vi "Setup UI.vi"(8 "error in (no error)":errorcluster, 11 "Operator UI in":refnum<class "Measurement UI.lvclass">) -> (0 "error out":errorcluster, 3 "Operator UI out":refnum<class "Measurement UI.lvclass">)   [LabVIEW 2015, in "Measurement UI.lvlib" / "Measurement UI.lvclass"]
uses:
  Measurement UI.lvclass
  Measurement UI.lvclass/Measurement UI.ctl
  <vilib>/Utility/miscctls.llb/LVRowAndColumnTypeDef.ctl
  <vilib>/Utility/miscctls.llb/LVRowAndColumnUnsignedTypeDef.ctl
  Accessors/Read Show FP_.vi
  Accessors/Read Status Display.vi
  Accessors/Read Digitizer.vi
  Accessors/Read Results Listbox.vi
  Accessors/Read View Results.vi
  Accessors/Read Function Generator.vi
  Accessors/Read Tab Control.vi
  Read Multimeter.vi
  Accessors/Read Run.vi
  Accessors/Read Measurement.vi
  Accessors/Read Power Supply.vi
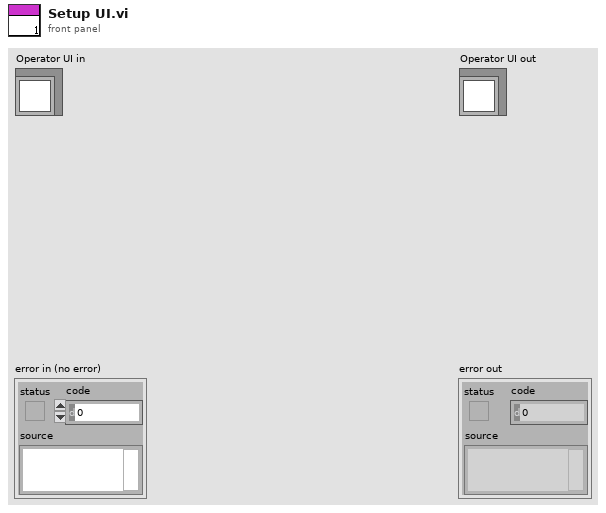
[diagram p1: front panel]
types:
  T1 = enum8{"Enabled", "Disabled", "Disabled and Grayed Out"}
  T2 = typedef "LVRowAndColumnUnsignedTypeDef.ctl" = cluster{"Row":u32, "Column":u32}
  T3 = typedef "LVRowAndColumnTypeDef.ctl" = cluster{"Row":i32, "Column":i32}
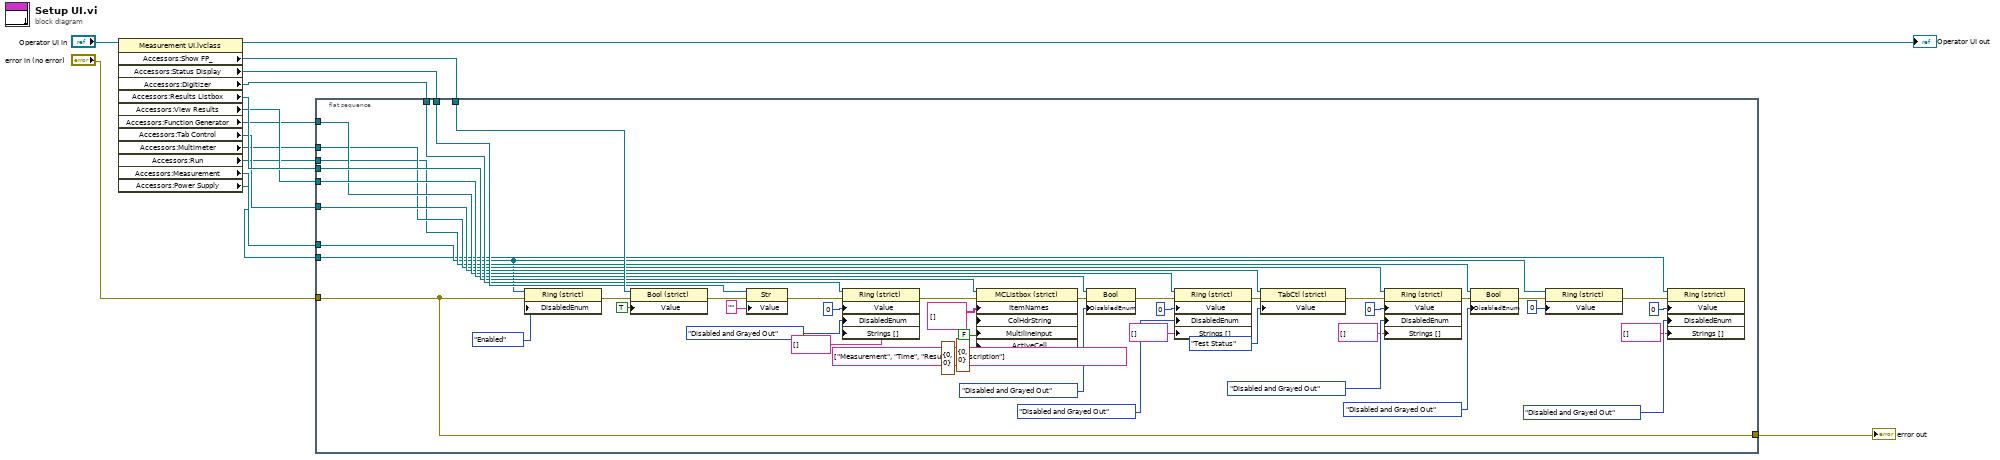
[diagram p0: block diagram]
diagram:
  n1 = property class="Measurement UI.lvclass"(reference="Operator UI in") -> (reference out=→"Operator UI out":refnum<class "Measurement UI.lvclass">, "Accessors:Show FP_"=w13:refnum<vi>, "Accessors:Status Display"=w12:refnum<vi>, "Accessors:Digitizer"=w11:refnum<vi>, "Accessors:Results Listbox"=w10:refnum<vi>, "Accessors:View Results"=w9:refnum<vi>, "Accessors:Function Generator"=w8:refnum<vi>, "Accessors:Tab Control"=w7:refnum<vi>, "Accessors:Multimeter"=w6:refnum<vi>, "Accessors:Run"=w5:refnum<vi>, "Accessors:Measurement"=w4:refnum<vi>, "Accessors:Power Supply"=w3:refnum<vi>)  [unwired: 1 in, 1 out]
  n2 = flat-sequence {
    tunnel: "error in (no error)" -> [w28]
    tunnel: [w28] -> w1
    tunnel: w13 -> [w26]
    tunnel: w12 -> [w25]
    tunnel: w11 -> [w24]
    tunnel: w10 -> [w23]
    tunnel: w9 -> [w22]
    tunnel: w8 -> [w21]
    tunnel: w7 -> [w20]
    tunnel: w6 -> [w19]
    tunnel: w5 -> [w18]
    tunnel: w4 -> [w17]
    tunnel: w3 -> [w16]
    frame #0 {
      n3 = property class="Ring (strict)"(reference=w17, error in=w28, "DisabledEnum"=T1."Enabled" ("Disabled")) -> (error out=w27:errorcluster)  [unwired: 1 out]
      n4 = property class="Bool (strict)"(reference=w26, error in=w27, "Value"=TRUE) -> (error out=w38:errorcluster)  [unwired: 1 out]
      n5 = property class="Str"(reference=w25, error in=w38, "Value"="") -> (error out=w39:errorcluster)  [unwired: 1 out]
      n6 = property class="Ring (strict)"(reference=w24, error in=w39, "Value"=u16 0, "DisabledEnum"=T1."Disabled and Grayed Out" ("Disabled"), "Strings []"=string[] []) -> (error out=w40:errorcluster)  [unwired: 1 out]
      n7 = property class="MCListbox (strict)"(reference=w23, error in=w40, "ItemNames"=string[][] [] ("Item Names"), "ColHdrString"=string[] ["Measurement", "Time", "Results", "Description"] ("Column Header Strings[]"), "MultilineInput"=FALSE ("Multiple Line Input"), "ActiveCell"=T3 {"Row"=0, "Column"=0} ("Active Cell:Active Cell"), "TopLeft"=T2 {"Row"=0, "Column"=0} ("Top Left Visible Cell")) -> (error out=w41:errorcluster)  [unwired: 1 out]
      n8 = property class="Bool"(reference=w22, error in=w41, "DisabledEnum"=T1."Disabled and Grayed Out" ("Disabled")) -> (error out=w42:errorcluster)  [unwired: 1 out]
      n9 = property class="Ring (strict)"(reference=w21, error in=w42, "Value"=u16 0, "DisabledEnum"=T1."Disabled and Grayed Out" ("Disabled"), "Strings []"=string[] []) -> (error out=w43:errorcluster)  [unwired: 1 out]
      n10 = property class="TabCtl (strict)"(reference=w20, error in=w43, "Value"=enum32{"Test Status", "Results"}."Test Status") -> (error out=w44:errorcluster)  [unwired: 1 out]
      n11 = property class="Ring (strict)"(reference=w19, error in=w44, "Value"=u16 0, "DisabledEnum"=T1."Disabled and Grayed Out" ("Disabled"), "Strings []"=string[] []) -> (error out=w45:errorcluster)  [unwired: 1 out]
      n12 = property class="Bool"(reference=w18, error in=w45, "DisabledEnum"=T1."Disabled and Grayed Out" ("Disabled")) -> (error out=w46:errorcluster)  [unwired: 1 out]
      n13 = property class="Ring (strict)"(reference=w17, error in=w46, "Value"=u16 0) -> (error out=w47:errorcluster)  [unwired: 1 out]
      n14 = property class="Ring (strict)"(reference=w16, error in=w47, "Value"=u16 0, "DisabledEnum"=T1."Disabled and Grayed Out" ("Disabled"), "Strings []"=string[] []) -> ()  [unwired: 2 out]
    }
  }
  "error out" <- w1
